vi "Module Cleanup.vi"(8 "error in (no error)":errorcluster, 11 "EStop Module in":refnum<class "EStop Module.lvclass">) -> (0 "error out":errorcluster, 3 "EStop Module out":refnum<class "EStop Module.lvclass">)   [LabVIEW 2020, in "VolatusControl.lvlib" / "EStop Module.lvclass"]
uses:
  EStop Module.lvclass
  EStop Module.lvclass/EStop Module.ctl
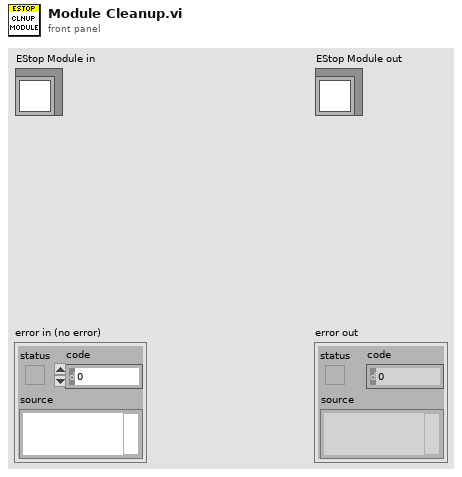
[diagram p1: front panel]
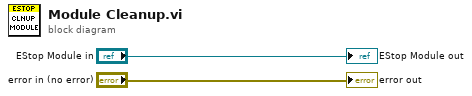
[diagram p0: block diagram]
diagram:
  "error out" <- "error in (no error)"
  "EStop Module out" <- "EStop Module in"
